vi "expect.vi"(8 "error in (no error)":errorcluster, 10 "data expected":string, 11 "TCP Network Connection in":refnum<k5>) -> (0 "error out":errorcluster, 2 "data read":string, 3 "TCP Network Connection out":refnum<k5>)   [LabVIEW 2020]
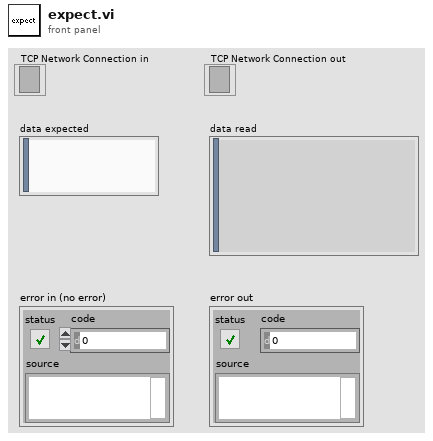
[diagram p1: front panel]
types:
  T1 = enum16{"Standard", "Buffered", "CRLF", "Immediate"}
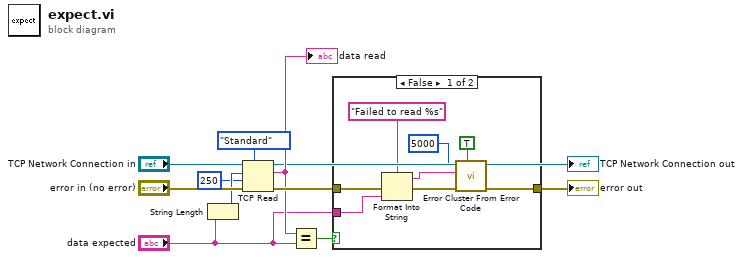
[diagram p0: block diagram]
diagram:
  n1 = String Length(string="data expected") -> (length=w2:i32)
  n2 = TCP Read(connection ID="TCP Network Connection in", bytes to read=w2, error in (no error)="error in (no error)", 7:T1."Standard" ("mode (standard)"), 9:250 ("timeout ms (25000)")) -> (connection ID out=→"TCP Network Connection out":refnum<k5>, data out=w8:string, error out=w11:errorcluster)
  "data read" <- w8
  n3 = Equal?(x=w8, y="data expected") -> (x = y?=w9:bool)
  n4 = case shown="False" w9 {
    tunnel: [w18 w20] -> w10
    tunnel: w11 -> [w19 w20]
    tunnel: "data expected" -> [w13 _]
    frame False {
      n5 = Format Into String(format string="Failed to read %s", error in=w19, w13) -> (resulting string=w12:string, error out=w15:errorcluster)  [unwired: 1 in]
      n6 = call <vilib>:"Error Cluster From Error Code.vi"("show call chain? (False)"=TRUE, "error in (no error)"=w15, "error message (\"\")"=w12, "error code (0)"=5000) -> ("error out"=w18:errorcluster)  [unwired: 5 in]
    }
    frame True {
    }
  }
  "error out" <- w10
